vi "TIMEOUT_SEND_CHECK_M114.vi"(8 "error IN":errorcluster, 9 "Serial Data Gcode":refnum<queue>, 10 "IN TIME":T1, 11 "STATE BOARD":enum16{"Running", "Waiting", "Pos", "IDLE"}(ring)) -> (0 "error out":errorcluster, 1 "OUT TIME":T1)   [LabVIEW 2017]
panel:
  in  "STEP SIZE":cluster{"X":dbl, "Y":dbl, "Z":dbl}
  in  "Max ACCEL":cluster{"X":dbl, "Y":dbl, "Z":dbl}
  in  "Max FEEDRATE":cluster{"X":dbl, "Y":dbl, "Z":dbl}
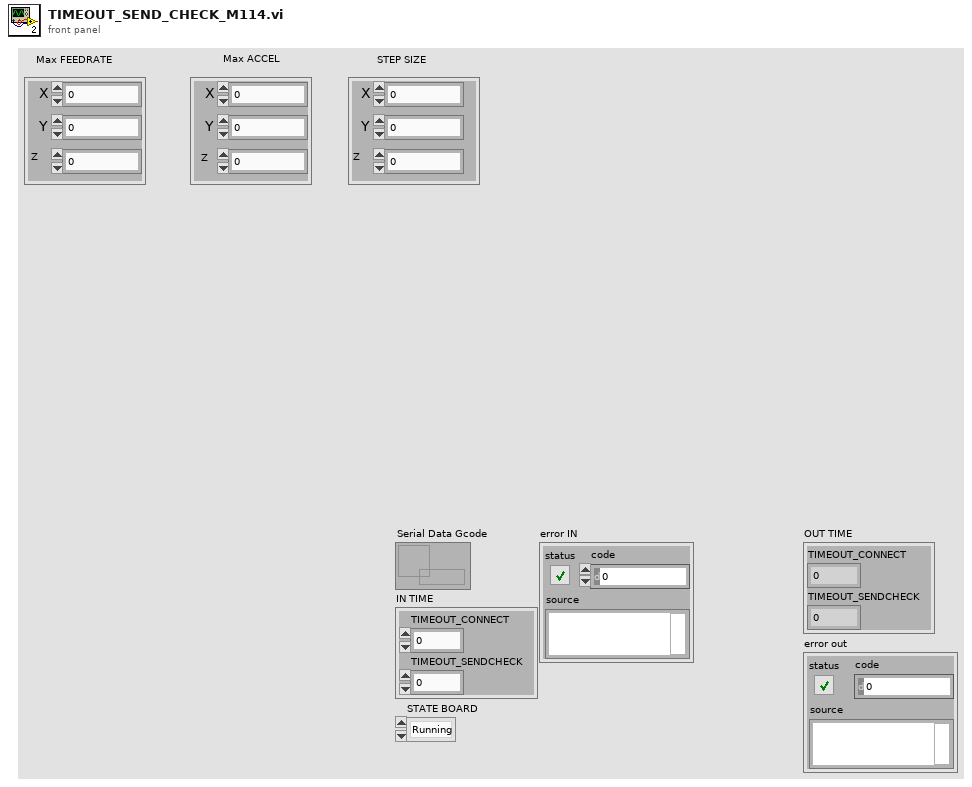
[diagram p1: front panel]
types:
  T1 = cluster{"TIMEOUT_CONNECT":u32, "TIMEOUT_SENDCHECK":u32}
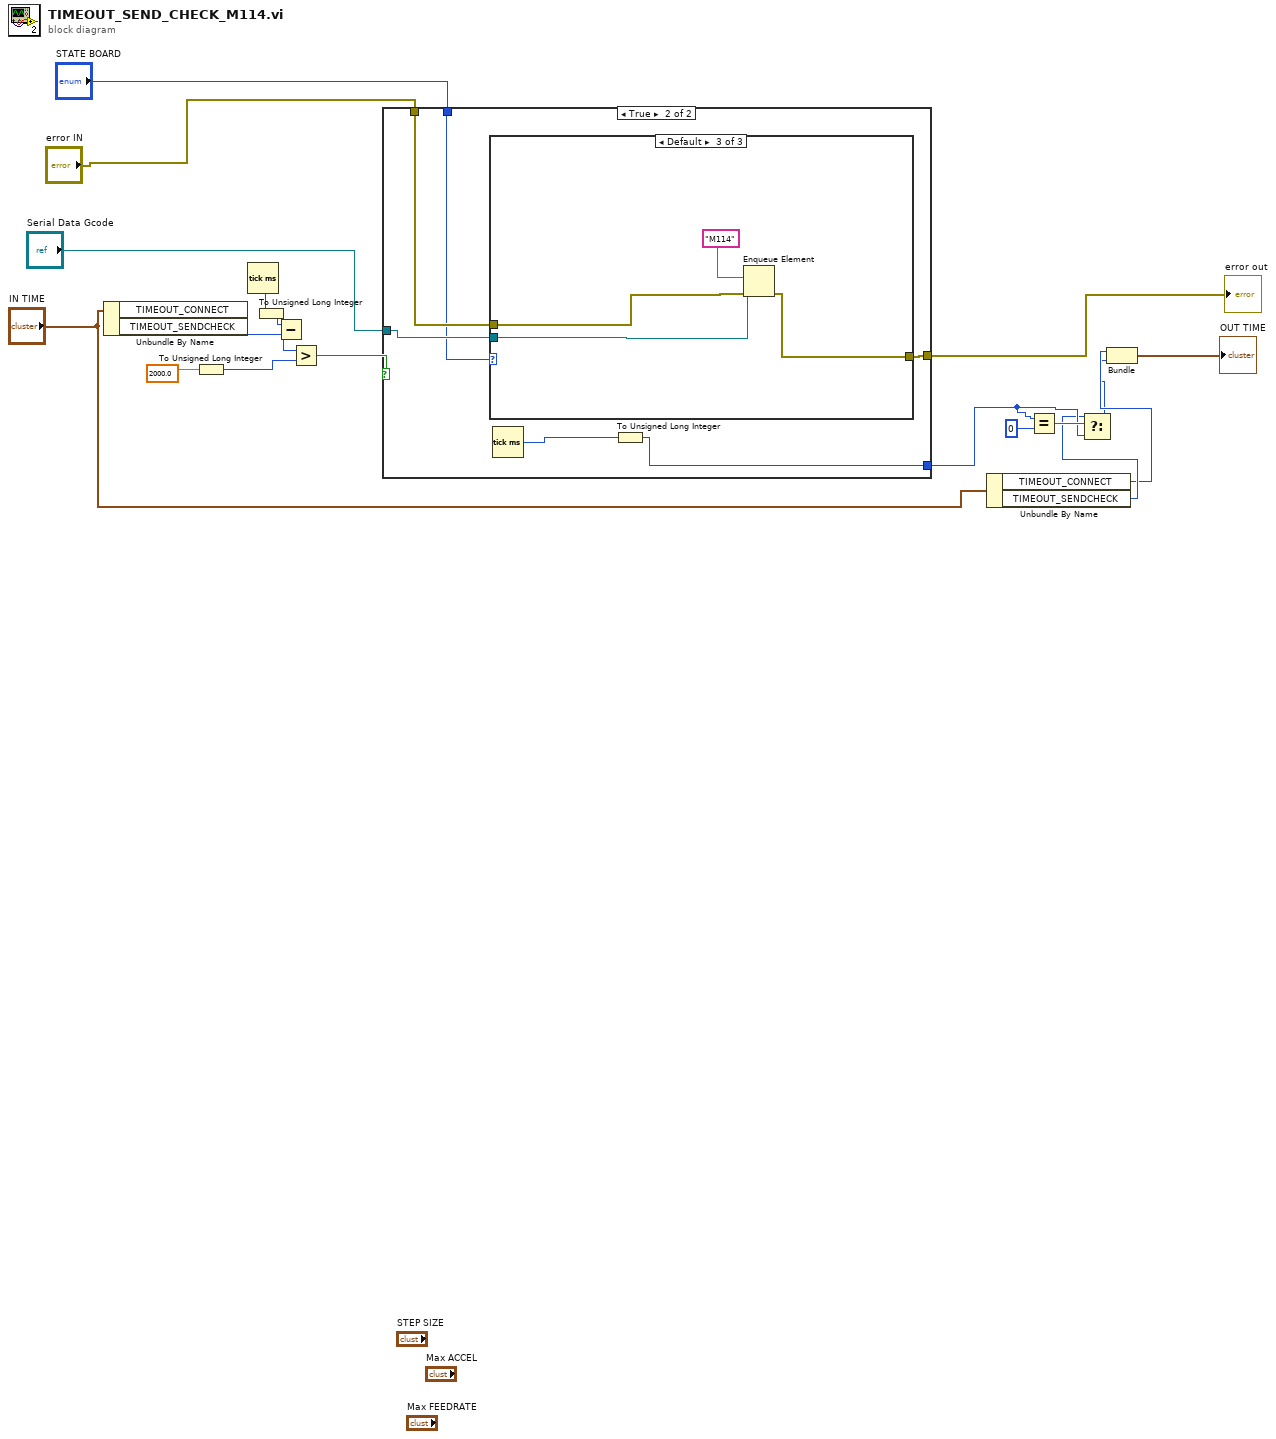
[diagram p0: block diagram]
diagram:
  n1 = Unbundle By Name("IN TIME") -> ("TIMEOUT_SENDCHECK"=w14:u32)  [unwired: 1 out]
  n2 = To Unsigned Long Integer(number=2000.0 ("y")) -> (unsigned 32bit integer=w16:u32)
  n3 = Tick Count (ms)() -> (millisecond timer value=w19:u32)
  n4 = To Unsigned Long Integer(number=w19) -> (unsigned 32bit integer=w18:u32)
  n5 = Subtract(x=w18, y=w14) -> (x-y=w17:u32)
  n6 = Greater?(x=w17, y=w16) -> (0:w13:bool)
  n7 = case shown="True" w13 {
    tunnel: [_ w26] -> w10
    tunnel: "Serial Data Gcode" -> [_ w23]
    tunnel: "error IN" -> [w20 w24]
    tunnel: [w20 w22] -> w3
    tunnel: "STATE BOARD" -> [_ w21]
    frame False {
    }
    frame True {
      n8 = case shown="Default" w21 {
        tunnel: w24 -> [_ _ w30]
        tunnel: w23 -> [_ _ w29]
        tunnel: [_ _ w28] -> w22
        frame "Running" {
        }
        frame "IDLE" {
        }
        frame Default {
          n9 = Enqueue Element(queue=w29, element="M114", error in (no error)=w30) -> (error out=w28:errorcluster)  [unwired: 1 in, 2 out]
        }
      }
      n10 = Tick Count (ms)() -> (millisecond timer value=w25:u32)
      n11 = To Unsigned Long Integer(number=w25) -> (unsigned 32bit integer=w26:u32)
    }
  }
  "error out" <- w3
  n12 = Unbundle By Name("IN TIME") -> ("TIMEOUT_CONNECT"=w8:u32, "TIMEOUT_SENDCHECK"=w9:u32)
  n13 = Equal?(x=w10, y=u32 0) -> (x = y?=w11:bool)
  n14 = Select(t=w9, s=w11, f=w10) -> (s? t:f=w7:u32)
  n15 = Bundle("TIMEOUT_CONNECT"=w8, "TIMEOUT_SENDCHECK"=w7) -> (→"OUT TIME":T1)  [unwired: 1 in]
